vi "GetCurrentMissionString.vi"() -> (1 "任务字符串":string)   [LabVIEW 2018]
panel:
  out "当前测量状态":T1(ring)
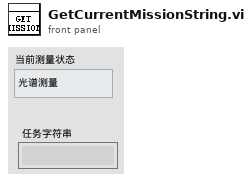
[diagram p1: front panel]
types:
  T1 = enum16{"光谱测量", "功率测量", "能量测量", "时间波形测量", "偏振测量", "近远场测量"}
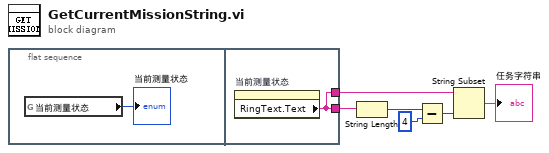
[diagram p0: block diagram]
diagram:
  n1 = flat-sequence {
    tunnel: [w8] -> w2
    tunnel: [w8] -> w1
    frame #0 {
      n2 = global read "参数.vi" "当前测量状态"() -> (→"当前测量状态":T1)
    }
    frame #1 {
      n3 = property on="当前测量状态" class="Enum (严格)"() -> ("RingText.Text"=w8:string)  [unwired: 2 in, 2 out]
    }
  }
  n4 = String Length(string=w1) -> (length=w6:i32)
  n5 = Subtract(x=w6, y=4) -> (x-y=w4:i32)
  n6 = String Subset(string=w2, length (rest)=w4) -> (substring=→"任务字符串":string)  [unwired: 1 in]
